vi "Math Marker Data.vi"(8 "error in (no error)":errorcluster, 9 "Marker Function (0: Flatness)":u16(ring) items=["Flatness", "RF Filter Statistics", "Statistics"], 10 "Channel (1)":i32=1, 11 "VISA resource name":refnum<visa-resource-name>) -> (0 "error out":errorcluster, 1 "Num3":dbl, 2 "Num2":dbl, 3 "VISA resource name out":refnum<visa-resource-name>, 4 "Num4":dbl, 5 "Num1":dbl)   [LabVIEW 2011, in "Agilent ENA Series.lvlib"]
doc: "For the active trace of channel, returns marker flatness or filter statistics or marker statistics data.\n\nNotes:\n(1) This VI is available only for ENA E5061A/E5062A."
uses:
  Agilent ENA Series.lvlib
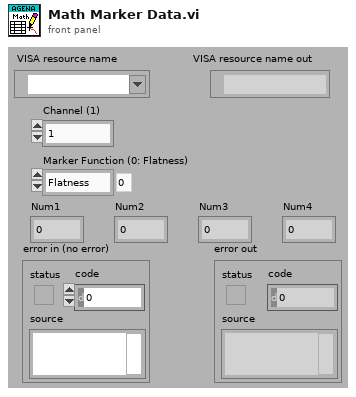
[diagram p1: front panel]
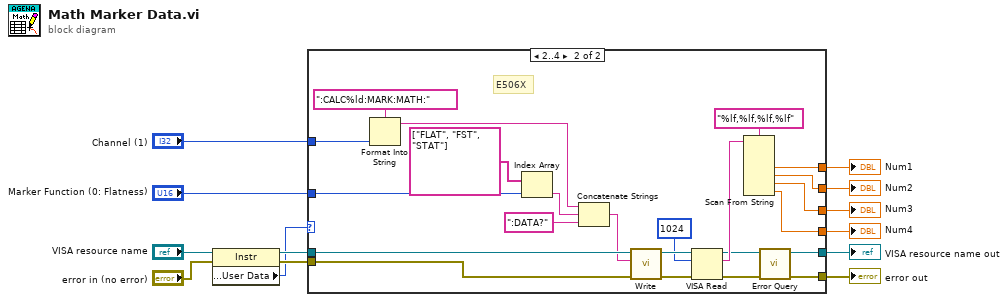
[diagram p0: block diagram]
diagram:
  n1 = property class="Instr"(reference="VISA resource name", error in="error in (no error)") -> (reference out=w9:refnum<visa-resource-name>, error out=w8:errorcluster, "General Settings:User Data"=w3:u32)
  n2 = case shown="2..4" w3 {
    tunnel: "Channel (1)" -> [_ w38]
    tunnel: "Marker Function (0: Flatness)" -> [_ w37]
    tunnel: w9 -> [w15 w36]
    tunnel: w8 -> [w14 w35]
    tunnel: [w15 w18] -> w2
    tunnel: [w14 w16] -> w1
    tunnel: [_ w28] -> w7
    tunnel: [_ w27] -> w6
    tunnel: [_ w26] -> w5
    tunnel: [_ w25] -> w4
    frame 0, Default {
    }
    frame 2..4 {
      # "E506X"
      n3 = Format Into String(format string=":CALC%ld:MARK:MATH:", w38) -> (resulting string=w20:string)  [unwired: 2 in, 1 out]
      n4 = Index Array(array=string[] ["FLAT", "FST", "STAT"], index=w37) -> (element=w21:string)
      n5 = Concatenate Strings(w20, w21, ":DATA?") -> (w34:string)
      n6 = call "Write.vi"("error in (no error)"=w35, "String ()"=w34, "VISA resource name"=w36) -> ("error out"=w32:errorcluster, "VISA resource name out"=w33:refnum<visa-resource-name>)  [unwired: 6 in, 1 out]
      n7 = VISA Read(VISA resource name=w33, byte count=u32 1024, error in (no error)=w32) -> (VISA resource name out=w19:refnum<visa-resource-name>, read buffer=w30:string, error out=w17:errorcluster)  [unwired: 1 out]
      n8 = Scan From String(format string="%lf,%lf,%lf,%lf", input string=w30) -> (output 1=w28:dbl, output 2=w27:dbl, output 3=w26:dbl, output 4=w25:dbl)  [unwired: 6 in, 3 out]
      n9 = call "Error Query.vi"("error in (no error)"=w17, "VISA resource name"=w19) -> ("error out"=w16:errorcluster, "VISA resource name out"=w18:refnum<visa-resource-name>)  [unwired: 6 in, 2 out]
    }
  }
  "VISA resource name out" <- w2
  "error out" <- w1
  "Num1" <- w7
  "Num2" <- w6
  "Num3" <- w5
  "Num4" <- w4
